vi "Test_WriteValue_InvalidRefnum_Error.vi"(8 "error in (no error)":errorcluster, 11 "TestCase in":refnum<class "TestTerminalValueBinding.lvclass">) -> (0 "error out":errorcluster, 3 "TestCase out":refnum<class "TestTerminalValueBinding.lvclass">)   [LabVIEW 2017, in "TestTerminalValueBinding.lvclass"]
uses:
  TestTerminalValueBinding.lvclass
  Source/Concrete/TerminalValueBinding/TerminalValueBinding.lvclass
  C:/Git/composed-transport/Source/ITransport/ITransport.lvclass
  Source/ITransport/ITransport.lvclass
panel:
  out "Return Error":errorcluster
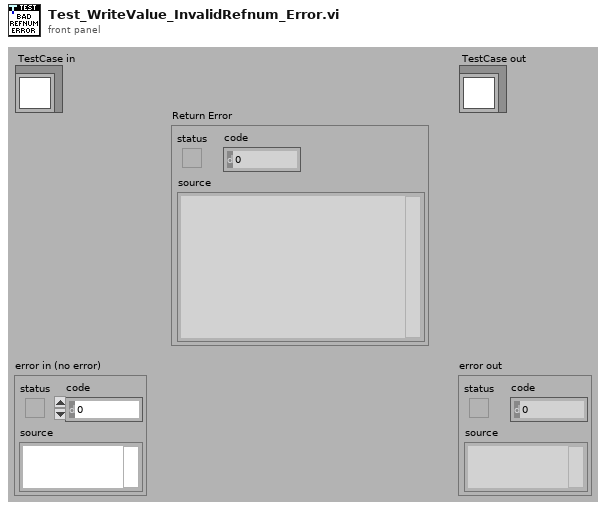
[diagram p1: front panel]
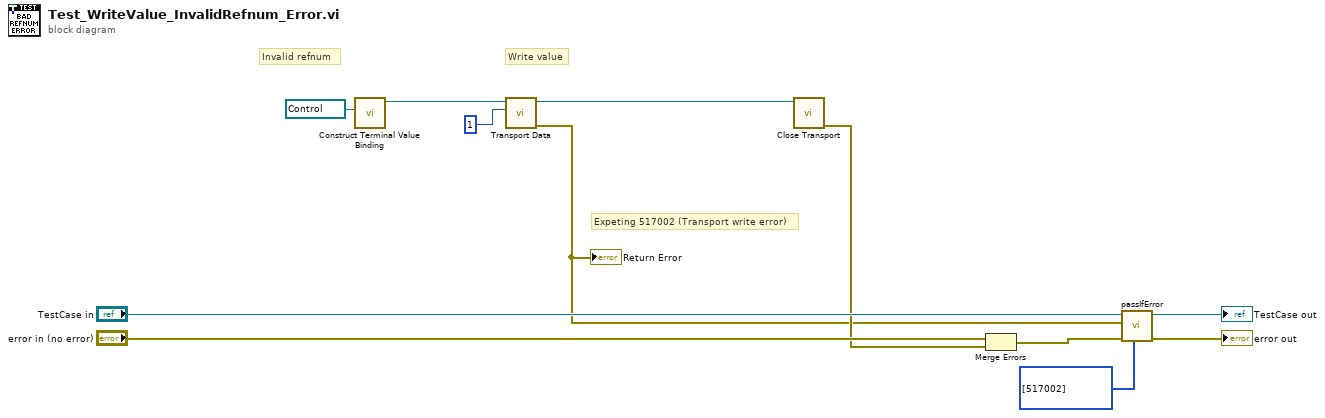
[diagram p0: block diagram]
diagram:
  # "Invalid refnum"
  # "Expeting 517002 (Transport write error)"
  # "Write value"
  n1 = call "Construct Terminal Value Binding.vi"("Ctl Refnum"=refnum<vi> refnum) -> ("TerminalValueBinding Out"=w8:refnum<class "TerminalValueBinding.lvclass">)  [unwired: 9 in, 1 out]
  n2 = call "Transport Data.vi"("Value"=1, "ITransport in"=w8) -> ("error out"=w3:errorcluster, "ITransport out"=w5:refnum<class "TerminalValueBinding.lvclass">)  [unwired: 8 in]
  "Return Error" <- w3
  n3 = call-dynamic "Close Transport.vi"("ITransport in"=w5) -> ("error out"=w4:errorcluster)  [unwired: 10 in]
  n4 = Merge Errors("error in (no error)", w4) -> (w7:errorcluster)
  n5 = call-dynamic "passIfError.vi"("passing error codes (default = any error code)"=i32[] [517002], "error in (no error)"=w7, "error"=w3, "TestCase in"="TestCase in") -> ("error out"=→"error out":errorcluster, "TestCase out"=→"TestCase out":refnum<class "TestTerminalValueBinding.lvclass">)  [unwired: 6 in]
